vi "Stop.vi"(8 "error in (no error)":errorcluster, 11 "Object ref in":T1) -> (0 "error out":errorcluster, 3 "Object ref out":T1)   [LabVIEW 2013, in "MaterialCharacterization.lvlib" / "MC-Main.lvclass"]
uses:
  MC-Main.lvclass
  Object-reference.ctl
  MC-Main.lvclass/MC-Main.ctl
  Application-status.ctl
  UI/Control-names.ctl
  Read UI.vi
  Read Status.vi
  UI/Set-control-enable-multiple.vi
  UI/MC-UI.lvclass
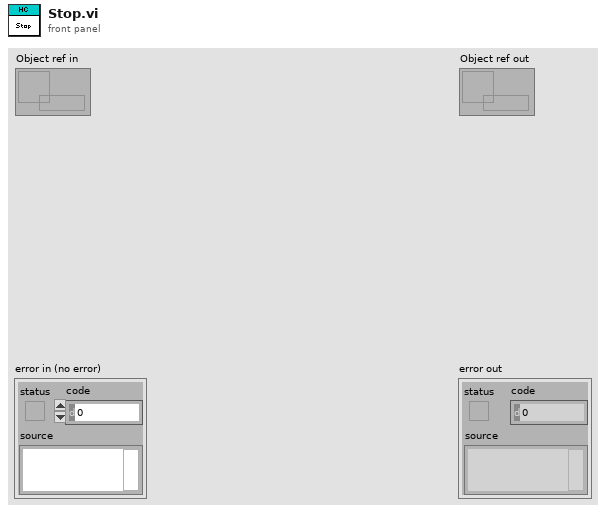
[diagram p1: front panel]
types:
  T1 = typedef "MaterialCharacterization.lvlib/MC-Main.lvclass/Object-reference.ctl" = refnum<data-value>
  T2 = typedef "MaterialCharacterization.lvlib/MC-Main.lvclass/Application-status.ctl" = enum16{"Idle", "Initialized", "Configured", "Activated", "Started", "Paused", "Stopped", "Reset", "Error", "Exited"}
  T3 = typedef "HardwareCharacterization.lvlib/HC-Main.lvclass/Application-status.ctl" = enum16{"Idle", "Initialized", "Configured", "Activated", "Started", "Paused", "Stopped", "Reset", "Error", "Exited"}
  T4 = typedef "MaterialCharacterization.lvlib/MC-UI.lvclass/Control-names.ctl" = enum16{"Help", "Status", "Load configuration", "Save configuration", "Activate", "Start", "Stop", "Options"}
  T5 = typedef "MaterialCharacterization.lvlib/MC-UI.lvclass/Panes-reference.ctl" = refnum<data-value>
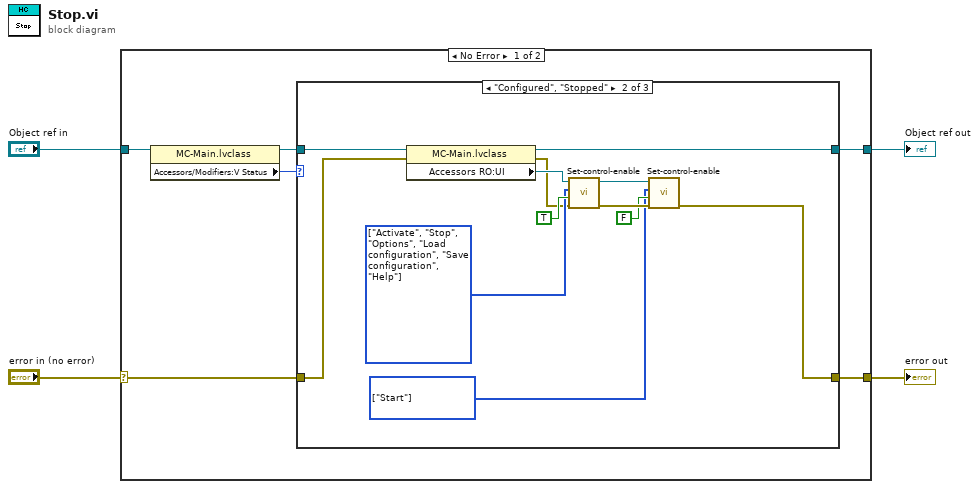
[diagram p0: block diagram]
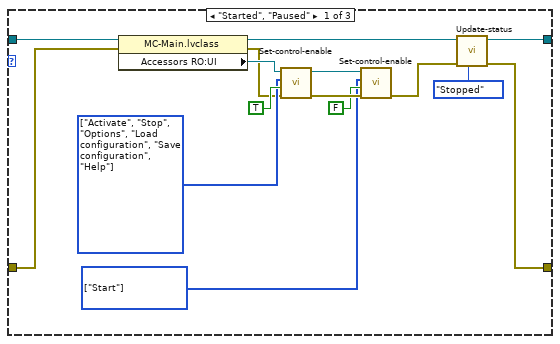
[diagram p2: hidden frame]
diagram:
  n1 = case shown="No Error" "error in (no error)" {
    selector: "error in (no error)" -> [w8 w41]
    tunnel: [w10 w41] -> w3
    tunnel: [w9 w40] -> w1
    tunnel: "Object ref in" -> [w7 w40]
    frame No Error {
      n2 = property class="MC-Main.lvclass"(reference=w7) -> (reference out=w6:T1, "Accessors/Modifiers:V Status"=w5:T3)  [unwired: 1 in, 1 out]
      n3 = case shown="\"Configured\", \"Stopped\"" w5 {
        tunnel: [w24 w27 w38] -> w10
        tunnel: [w23 w26 w39] -> w9
        tunnel: w6 -> [w14 w29 w39]
        tunnel: w8 -> [w13 w28 w38]
        frame "Started", "Paused" {
          w15 = T4[] [enum."Start"] items=["Help", "Status", "Load configuration", "Save configuration", "Activate", "Start", "Stop", "Options"] ("Control names")
          w20 = T4[] [enum."Activate", enum."Stop", enum."Options", enum."Load configuration", enum."Save configuration", enum."Help"] items=["Help", "Status", "Load configuration", "Save configuration", "Activate", "Start", "Stop", "Options"] ("Control names")
          n4 = property class="MC-Main.lvclass"(reference=w14, error in=w13) -> (reference out=w11:T1, error out=w19:errorcluster, "Accessors RO:UI"=w21:T5)
          n5 = call-poly "Set-control-enable.vi"("error in (no error)"=w19, "Enable?"=TRUE, "Control names"=w20, "Panes in"=w21) -> ("error out"=w17:errorcluster, "Panes out"=w18:T5)  [unwired: 6 in]
          n6 = call-poly "Set-control-enable.vi"("error in (no error)"=w17, "Enable?"=FALSE, "Control names"=w15, "Panes in"=w18) -> ("error out"=w12:errorcluster)  [unwired: 6 in, 1 out]
          n7 = call "Update-status.vi"("Status"=Application-status."Stopped", "error in (no error)"=w12, "Object ref in"=w11) -> ("error out"=w24:errorcluster, "Object ref out"=w23:T1)  [unwired: 7 in]
        }
        frame "Configured", "Stopped" {
          w30 = T4[] [enum."Start"] items=["Help", "Status", "Load configuration", "Save configuration", "Activate", "Start", "Stop", "Options"] ("Control names")
          w35 = T4[] [enum."Activate", enum."Stop", enum."Options", enum."Load configuration", enum."Save configuration", enum."Help"] items=["Help", "Status", "Load configuration", "Save configuration", "Activate", "Start", "Stop", "Options"] ("Control names")
          n8 = property class="MC-Main.lvclass"(reference=w29, error in=w28) -> (reference out=w26:T1, error out=w34:errorcluster, "Accessors RO:UI"=w36:T5)
          n9 = call-poly "Set-control-enable.vi"("error in (no error)"=w34, "Enable?"=TRUE, "Control names"=w35, "Panes in"=w36) -> ("error out"=w32:errorcluster, "Panes out"=w33:T5)  [unwired: 6 in]
          n10 = call-poly "Set-control-enable.vi"("error in (no error)"=w32, "Enable?"=FALSE, "Control names"=w30, "Panes in"=w33) -> ("error out"=w27:errorcluster)  [unwired: 6 in, 1 out]
        }
        frame Default {
        }
      }
    }
    frame Error {
    }
  }
  "error out" <- w3
  "Object ref out" <- w1
